vi "liblinear_train.vi"(8 "error in (no error)":errorcluster, 10 "parameters":T2={"solver_type"=0, "eps"=0.01, "C"=1.0, "weight_label"=[], "weight"=[], "p"=0.1} {"solver_type" items=["L2R_LR"=0, "L2R_L2LOSS_SVC_DUAL"=1, "L2R_L2LOSS_SVC"=2, "L2R_L1LOSS_SVC_DUAL"=3, "MCSVM_CS"=4, "L1R_L2LOSS_SVC"=5, "L1R_LR"=6, "L2R_LR_DUAL"=7, "L2R_L2LOSS_SVR"=11, "L2R_L2LOSS_SVR_DUAL"=12, "L2R_L1LOSS_SVR_DUAL"=13]}, 11 "problem":T4={"y"=[], "x"=[], "bias"=-1.0}) -> (0 "error out":errorcluster, 3 "model":T1={"liblinear_parameter"={"solver_type"=0, "eps"=0.01, "C"=1.0, "weight_label"=[], "weight"=[], "p"=0.1}, "nr_class"=0, "nr_feature"=0, "w"=[], "label"=[], "bias"=0.0} {"liblinear_parameter"."solver_type" items=["L2R_LR"=0, "L2R_L2LOSS_SVC_DUAL"=1, "L2R_L2LOSS_SVC"=2, "L2R_L1LOSS_SVC_DUAL"=3, "MCSVM_CS"=4, "L1R_L2LOSS_SVC"=5, "L1R_LR"=6, "L2R_LR_DUAL"=7, "L2R_L2LOSS_SVR"=11, "L2R_L2LOSS_SVR_DUAL"=12, "L2R_L1LOSS_SVR_DUAL"=13]})   [LabVIEW 2015]
uses:
  Controls/liblinear_problem.ctl
  LibSVM Sparse/Wrapper API/Controls/svm_node.ctl
  Controls/liblinear_parameter.ctl
  Controls/liblinear_solver.ctl
  Controls/liblinear_model.ctl
  bin/x64/LabVIEW-liblinear.dll
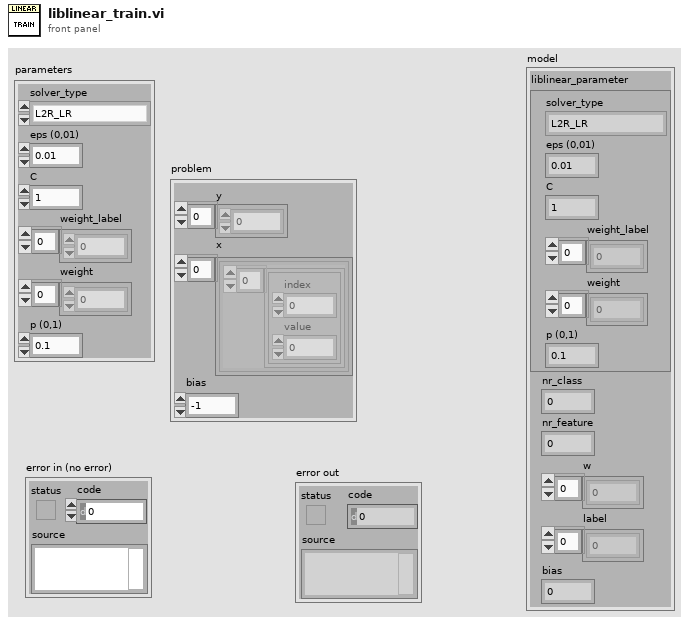
[diagram p1: front panel]
types:
  T1 = typedef "liblinear_model.ctl" = cluster{"liblinear_parameter":T2, "nr_class":i32, "nr_feature":i32, "w":dbl[], "label":i32[], "bias":dbl}
  T2 = typedef "liblinear_parameter.ctl" = cluster{"solver_type":T3, "eps":dbl, "C":dbl, "weight_label":i32[], "weight":dbl[], "p":dbl}
  T3 = typedef "liblinear_solver.ctl" = u32
  T4 = typedef "liblinear_problem.ctl" = cluster{"y":dbl[], "x":cluster{T5[]}[], "bias":dbl}
  T5 = typedef "svm_node.ctl" = cluster{"index":i32, "value":dbl}
  T6 = typedef "liblinear_problem_padded.ctl" = cluster{"y":dbl[], "x":cluster{T7[]}[], "bias":dbl}
  T7 = typedef "svm_node_padded.ctl" = cluster{"index":i32, "padding":i32, "value":dbl}
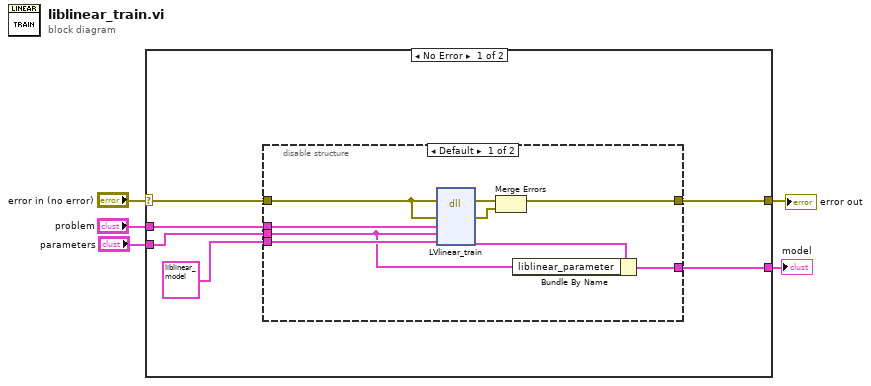
[diagram p0: block diagram]
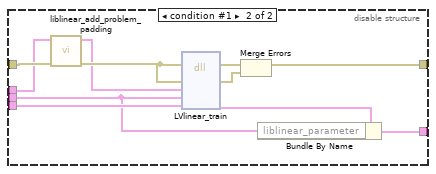
[diagram p2: hidden frame]
diagram:
  n1 = case shown="No Error" "error in (no error)" {
    selector: "error in (no error)" -> [w11 w32]
    tunnel: [w10 w32] -> w5
    tunnel: "problem" -> [w9 _]
    tunnel: "parameters" -> [w7 _]
    tunnel: [w6 _] -> w1
    frame No Error {
      n2 = disable-structure shown="Default" {
        disable-tunnel: w11 -> [w20 w24]
        disable-tunnel: [w17 w29] -> w10
        disable-tunnel: w9 -> [w16 w22]
        disable-tunnel: T1 {"liblinear_parameter"={"solver_type"=0, "eps"=0.01, "C"=1.0, "weight_label"=[], "weight"=[], "p"=0.1}, "nr_class"=0, "nr_feature"=0, "w"=[], "label"=[], "bias"=0.0} ("liblinear_model") -> [w15 w28]
        disable-tunnel: w7 -> [w13 w26]
        disable-tunnel: [w12 w25] -> w6
        frame condition #0 (active) {
          n3 = dll-call lib="C:/dev/LabVIEW-libsvm/LabVIEW/bin/x64/LabVIEW-liblinear.dll" fn="LVlinear_train"(error in=w20, "lvErr"=w20, "prob_in"=w16, "param_in"=w13, "model_out"=w15) -> (error out=w19:errorcluster, "lvErr"=w18:errorcluster, "model_out"=w14:T1)  [unwired: 5 in, 1 out]
          n4 = Merge Errors(w19, w18) -> (w17:errorcluster)
          n5 = Bundle By Name(cluster=w14, "liblinear_parameter"=w13) -> (w12:T1)
        }
        frame condition #1 {
          n6 = call "liblinear_add_problem_padding.vi"("error in (no error)"=w24, "problem"=w22) -> ("error out"=w23:errorcluster, "problem padded"=w21:T6)  [unwired: 8 in]
          n7 = dll-call lib="C:/dev/LabVIEW-libsvm/LabVIEW/bin/x64/LabVIEW-liblinear.dll" fn="LVlinear_train"(error in=w23, "lvErr"=w23, "prob_in"=w21, "param_in"=w26, "model_out"=w28) -> (error out=w31:errorcluster, "lvErr"=w30:errorcluster, "model_out"=w27:T1)  [unwired: 5 in, 1 out]
          n8 = Merge Errors(w31, w30) -> (w29:errorcluster)
          n9 = Bundle By Name(cluster=w27, "liblinear_parameter"=w26) -> (w25:T1)
        }
      }
    }
    frame Error {
    }
  }
  "error out" <- w5
  "model" <- w1
